vi "Calc From To Deltas.vi"(7 "Texture Dimensions":T1, 9 "Steps":i32, 10 "To":T2 {"v" min=0 max=1 step=0.1; "u" min=0 max=1 step=0.1}, 11 "From":T2 {"v" min=0 max=1 step=0.1; "u" min=0 max=1 step=0.1}) -> (3 "Deltas (Texels Per Step)":T2 {"v" min=0 max=1 step=0.1; "u" min=0 max=1 step=0.1})   [LabVIEW 2022 SP3, in "Raster.lvlib"]
uses:
  Raster.lvlib
  UV.ctl
  Rectangle Dimensions.ctl
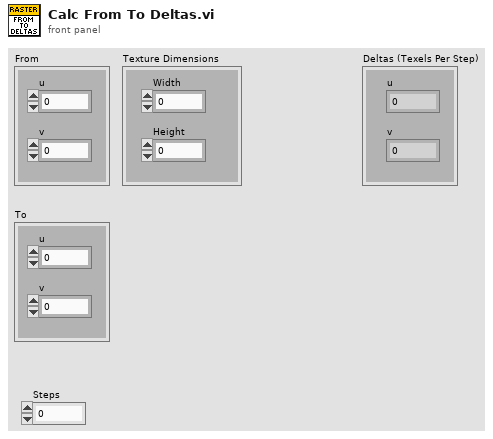
[diagram p1: front panel]
types:
  T1 = typedef "Raster.lvlib/Rectangle Dimensions.ctl" = cluster{"Width":u32, "Height":u32}
  T2 = typedef "Raster.lvlib/UV.ctl" = cluster{"u":sgl, "v":sgl}
  T3 = typedef "Raster.lvlib/Point 2D (SGL).ctl" = cluster{"x":sgl, "y":sgl}
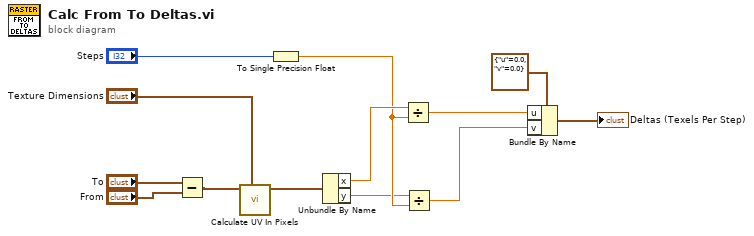
[diagram p0: block diagram]
diagram:
  n1 = Subtract(x="To", y="From") -> (x-y=w7:T2)
  n2 = call "Calculate UV In Pixels.vi"("Texture Dimensions"="Texture Dimensions", "UV"=w7) -> ("Pixels"=w1:T3)  [unwired: 9 in]
  n3 = To Single Precision Float(number="Steps") -> (single precision float=w10:sgl)
  n4 = Unbundle By Name(w1) -> ("x"=w11:sgl, "y"=w9:sgl)
  n5 = Divide(x=w11, y=w10) -> (x/y=w12:sgl)
  n6 = Divide(x=w9, y=w10) -> (x/y=w13:sgl)
  n7 = Bundle By Name(cluster=T2 {"u"=0.0, "v"=0.0} ("Start Deltas"), "u"=w12, "v"=w13) -> (→"Deltas (Texels Per Step)":T2)
